vi "Measurement selected.vi"(8 "error in (no error)":errorcluster, 10 "Coords":T1, 11 "ZenGage v3.0 UI in":refnum<class "ZenGage v3.0 UI.lvclass">) -> (0 "error out":errorcluster, 3 "ZenGage v3.0 UI out":refnum<class "ZenGage v3.0 UI.lvclass">)   [LabVIEW 2015, in "ZenGage v3.0 UI.lvclass"]
uses:
  ZenGage v3.0 UI.lvclass
  <vilib>/Utility/miscctls.llb/LVPoint32TypeDef.ctl
  ZenGage v3.0 UI.lvclass/ZenGage v3.0 UI.ctl
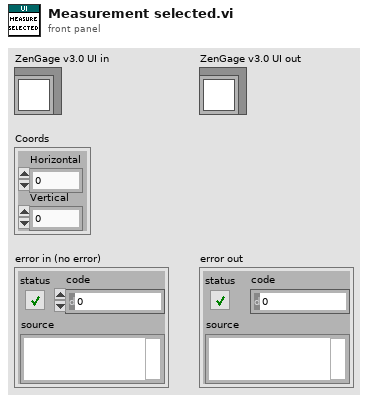
[diagram p1: front panel]
types:
  T1 = typedef "LVPoint32TypeDef.ctl" = cluster{"Horizontal":i32, "Vertical":i32}
  T2 = typedef "ZenGage v3.0 UI.lvclass/Edit Tolerance Input.ctl" = cluster{"ETL controls":T3, "Input Data Cluster":cluster{"Measurement Values":string[][], "Cluster of Limits":cluster{"LSL":dbl, "USL":dbl, "LCL":dbl, "UCL":dbl}, "Rack Selection":T4, "M and N Array":cluster{"M1":u64, "M2":u64, "N1":u64, "N2":u64}[], "Ticked Measurement Index":u32[], "Measurements Enabled":bool[], "Current Active Position":T1, "Current ticked measurement":dbl}}
  T3 = typedef "ETL controls.ctl" = cluster{"Measurement\n ListBox":refnum<vi>, "Cluster of limits":refnum<vi>, "Thresholds limits":refnum<vi>, "Bias Correction":refnum<vi>, "Linearity Correction":refnum<vi>}
  T4 = typedef "ZenGage v3.0 UI.lvclass/Rack Selection.ctl" = enum16{"Both Racks", "Rack 2", "Rack 1"}
  T5 = enum8{"Enabled", "Disabled", "Disabled and Grayed Out"}
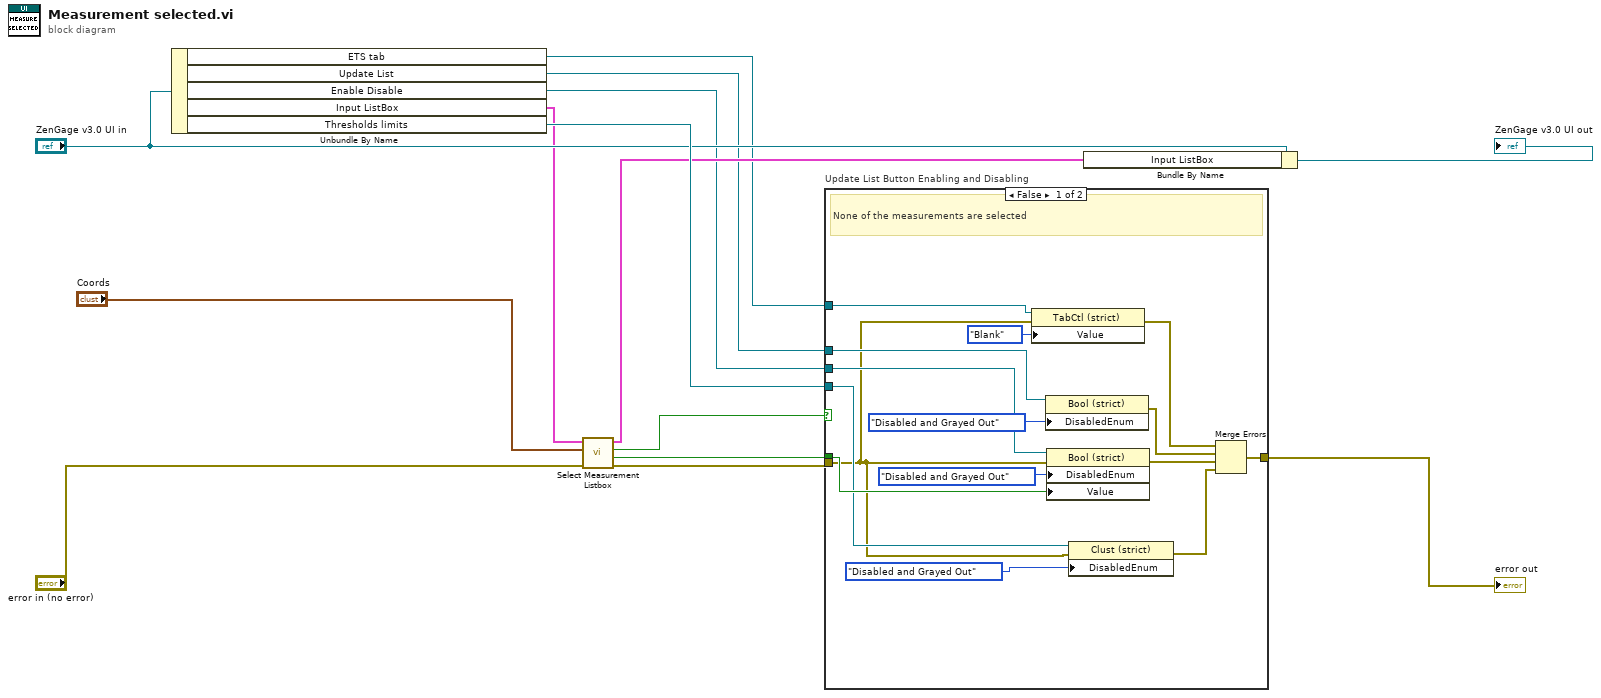
[diagram p0: block diagram]
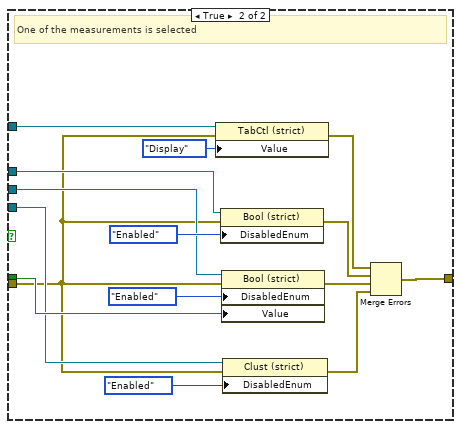
[diagram p2: hidden frame]
diagram:
  n1 = Unbundle By Name("ZenGage v3.0 UI in") -> ("ETS tab"=w1:refnum<vi>, "Update List"=w4:refnum<vi>, "Enable Disable"=w5:refnum<vi>, "Input ListBox"=w9:T2, "Thresholds limits"=w14:refnum<vi>)
  n2 = call "Select Measurement Listbox.vi"("error in (no error)"="error in (no error)", "Coords"="Coords", "Input ListBox in"=w9) -> ("error out"=w3:errorcluster, "Enable Disable button state"=w7:bool, "Tick Marked?"=w6:bool, "ListBox Cluster out"=w11:T2)  [unwired: 5 in]
  n3 = case "Update List Button Enabling and Disabling" shown="False" w6 {
    tunnel: w4 -> [w29 w44]
    tunnel: [w24 w39] -> w8
    tunnel: w7 -> [w23 w38]
    tunnel: w3 -> [w15 w30]
    tunnel: w5 -> [w22 w37]
    tunnel: w14 -> [w21 w35]
    tunnel: w1 -> [w18 w32]
    frame False {
      # "None of the measurements are selected"
      n4 = property class="TabCtl (strict)"(reference=w18, error in=w15, "Value"=enum32{"Display", "Blank"}."Blank") -> (error out=w16:errorcluster)  [unwired: 1 out]
      n5 = property class="Bool (strict)"(reference=w29, "DisabledEnum"=T5."Disabled and Grayed Out" ("Disabled")) -> (error out=w25:errorcluster)  [unwired: 1 in, 1 out]
      n6 = property class="Bool (strict)"(reference=w22, error in=w15, "DisabledEnum"=T5."Disabled and Grayed Out" ("Disabled"), "Value"=w23) -> (error out=w26:errorcluster)  [unwired: 1 out]
      n7 = property class="Clust (strict)"(reference=w21, error in=w15, "DisabledEnum"=T5."Disabled and Grayed Out" ("Disabled")) -> (error out=w20:errorcluster)  [unwired: 1 out]
      n8 = Merge Errors(w16, w25, w26, w20) -> (w24:errorcluster)
    }
    frame True {
      # "One of the measurements is selected"
      n9 = property class="TabCtl (strict)"(reference=w32, error in=w30, "Value"=enum32{"Display", "Blank"}."Display") -> (error out=w33:errorcluster)  [unwired: 1 out]
      n10 = property class="Bool (strict)"(reference=w44, error in=w30, "DisabledEnum"=T5."Enabled" ("Disabled")) -> (error out=w40:errorcluster)  [unwired: 1 out]
      n11 = property class="Bool (strict)"(reference=w37, error in=w30, "DisabledEnum"=T5."Enabled" ("Disabled"), "Value"=w38) -> (error out=w41:errorcluster)  [unwired: 1 out]
      n12 = property class="Clust (strict)"(reference=w35, error in=w30, "DisabledEnum"=T5."Enabled" ("Disabled")) -> (error out=w36:errorcluster)  [unwired: 1 out]
      n13 = Merge Errors(w33, w40, w41, w36) -> (w39:errorcluster)
    }
  }
  "error out" <- w8
  n14 = Bundle By Name(cluster="ZenGage v3.0 UI in", "Input ListBox"=w11) -> (→"ZenGage v3.0 UI out":refnum<class "ZenGage v3.0 UI.lvclass">)
